vi "Write UI Ref.vi"(8 "error in (no error)":errorcluster, 10 "UI Ref":refnum<vi>, 11 "Analyze Results Energy in":refnum<class "Analyze Results Energy.lvclass">) -> (0 "error out":errorcluster, 3 "Analyze Results Energy out":refnum<class "Analyze Results Energy.lvclass">)   [LabVIEW 2014, in "Analyze Results Energy.lvclass"]
uses:
  Analyze Results Energy.lvclass
  Analyze Results Energy.lvclass/Analyze Results Energy.ctl
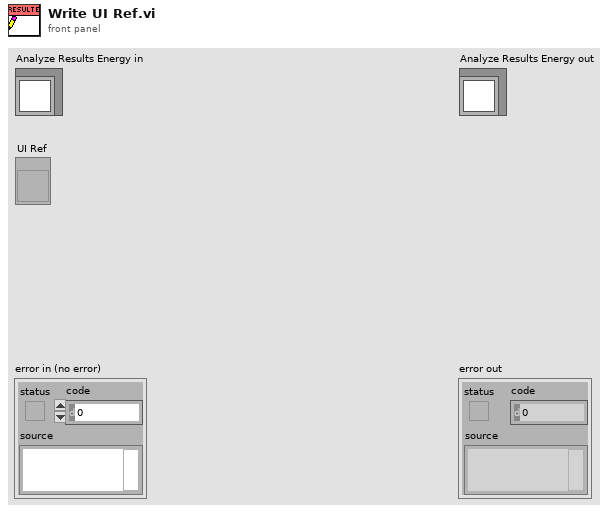
[diagram p1: front panel]
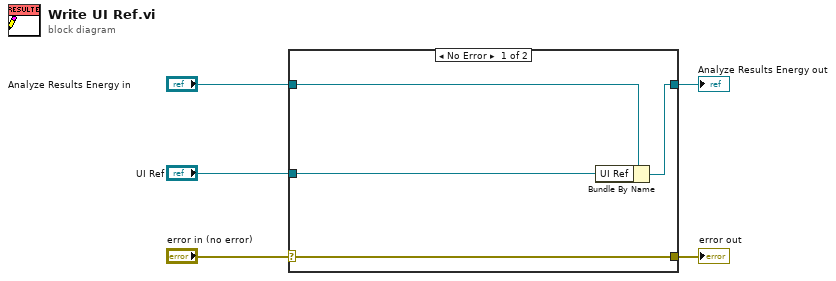
[diagram p0: block diagram]
diagram:
  n1 = case shown="No Error" "error in (no error)" {
    selector: "error in (no error)" -> [w9 w10]
    tunnel: [w9 w10] -> w4
    tunnel: [w7 w11] -> w2
    tunnel: "Analyze Results Energy in" -> [w8 w11]
    tunnel: "UI Ref" -> [w6 _]
    frame No Error {
      n2 = Bundle By Name(cluster=w8, "UI Ref"=w6) -> (w7:refnum<class "Analyze Results Energy.lvclass">)
    }
    frame Error {
    }
  }
  "error out" <- w4
  "Analyze Results Energy out" <- w2
